vi "Bool_Edge Detect.vi"(9 "Initial State":bool, 11 "Input/Set":bool) -> (0 "Change":bool, 1 "Fall":bool, 2 "Rise":bool, 3 "Output":bool)   [LabVIEW 2023]
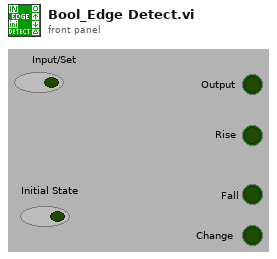
[diagram p1: front panel]
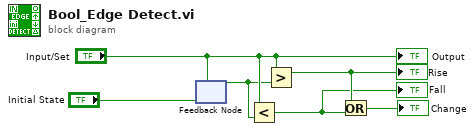
[diagram p0: block diagram]
diagram:
  n1 = feedback-in #1("Input/Set") -> ()
  n2 = feedback #1("Initial State") -> (w4:bool)
  n3 = Less?(x="Input/Set", y=w4) -> (x < y?=w2:bool)
  "Fall" <- w2
  n4 = Greater?(x="Input/Set", y=w4) -> (0:w3:bool)
  "Rise" <- w3
  n5 = Or(x=w3, y=w2) -> (x .or. y?=→"Change":bool)
  "Output" <- "Input/Set"
